vi "Catapult Loop.vi"   [LabVIEW 2015]
uses:
  Robot Global Data.vi
  <vilib>/Rock Robotics/WPI/Solenoid/Deprecated/WPI_SolenoidSetBool.vi
types:
  T1 = typedef "Dashboard Control Data.ctl" = cluster{"Encoder Control":T2, "Steer PID output":cluster{"output high":dbl, "output low":dbl}, " Steer PID gains":cluster{"proportional gain (Kc)":dbl, "integral time (Ti, min)":dbl, "derivative time (Td, min)":dbl}, "Drivetrain Settings":T3, "Vision Packet":T4, "Dashboard Drivetrain Command":T5, "Info/Command Cluster":T7, "Ball Vision Packet":T8, "Intake Presets":T10, "Intake Encoder Control":T12, "Climb Presets":T13, "Goal Output Range":cluster{"output high":dbl, "output low":dbl}, "Enabled Systems":T14, "Auton Presets":T15, "Pressure M":dbl, "Pressure B":dbl, "Vision Timeout":dbl, "Auto-Shift":T16, "Catapult Setpoints":T17}
  T2 = typedef "Encoder Control.ctl" = cluster{"Right Tick Constant":dbl, "Left Tick Constant":dbl, "Reset?":bool, "Y Dist":cluster{"PID gains":cluster{"proportional gain (Kc)":dbl, "integral time (Ti, min)":dbl, "derivative time (Td, min)":dbl}}, "Y Stop Thresh":dbl, "Y Stop Speed":dbl}
  T3 = typedef "Drivetrain Settings.ctl" = cluster{"Gyro Tolerance":dbl, "Throttle Ramp (ms)":dbl, "Kv":dbl, "Ka":dbl, "Feed Forward P":dbl, "Feed Forward D":dbl, "Goal Vision PID gains":cluster{"proportional gain (Kc)":dbl, "integral time (Ti, min)":dbl, "derivative time (Td, min)":dbl}, "Goal Detection Window":dbl, "Creep Rate":dbl, "Vision Throttle Threshold":dbl, "Min Turn Output":dbl, "Left Batter Angle":dbl, "Right Batter Angle":dbl}
  T4 = typedef "Goal Vision Packet.ctl" = cluster{"Distance":dbl, "Center X":dbl, "Center Y":dbl, "Found Target?":bool, "Robot Center":dbl, "Angle":dbl}
  T5 = typedef "Dashboard Drivetrain Command.ctl" = cluster{"Drivetrain Vision":T6}
  T6 = typedef "Drivetrain Vision.ctl" = cluster{"Goal Window":dbl, "Ball Window":dbl}
  T7 = typedef "Ball Tracking Command Cluster.ctl" = cluster{"Distance to Ball":dbl, "Desired Angle":dbl, "Command":enum16{"Turn to Ball", "Turn to Angle", "Get Distance"}, "Pixels from Center":dbl}
  T8 = typedef "Ball Vision Packet.ctl" = cluster{"Ball Detected?":bool, "Distance to Ball":dbl, "Desired Angle":dbl, "Pixels from Center":dbl, "Tracking mode":T9}
  T9 = typedef "Tracking Mode.ctl" = enum16{"Turn to Ball", "Turn to Angle"}
  T10 = typedef "Intake Presets.ctl" = cluster{"Intake Speed":dbl, "Outake Speed":dbl, "Low Height":dbl, "Half Height":dbl, "High Idle Height":dbl, "Angle Speed":dbl, "Angle Tolerance":dbl, "Encoder Scale":dbl, "Load Height":dbl, "Output Range":T11, "Rotation Power Max/Min":dbl, "MaxCurrent":dbl, "Intake Trip Time":dbl, "Idle Height":dbl, "Max Height":dbl, "Reset Encoders?":bool, "PID gains":cluster{"proportional gain (Kc)":dbl, "integral time (Ti, min)":dbl, "derivative time (Td, min)":dbl}, "Intake Stop Delay":u32, "Settle Time":dbl, "Settle Wait Time":dbl, "Pull Up Delay":dbl}
  T11 = typedef "Drivetrain Output Range.ctl" = cluster{"output high":dbl, "output low":dbl}
  T12 = typedef "IntakeEcoderControl.ctl" = cluster{"Arm Tick Constant":dbl, "Reset?":bool, "Y Dist":cluster{"PID gains":cluster{"proportional gain (Kc)":dbl, "integral time (Ti, min)":dbl, "derivative time (Td, min)":dbl}}, "Y Stop Thresh":dbl, "Y Stop Speed":dbl}
  T13 = typedef "Climb Presets.ctl" = cluster{"Pull Power":dbl, "Extend Power":dbl}
  T14 = typedef "Enabled Systems.ctl" = cluster{"Shoot":bool, "Intake":bool, "DT":bool, "Gyro":bool, "100ms":bool, "US":bool}
  T15 = typedef "Autonomous Presets.ctl" = cluster{"Pitch Limit":dbl, "Roll Limit":dbl, "Start Position":dbl, "Cross Position":dbl}
  T16 = typedef "Auto Shift Cluster.ctl" = cluster{"Delay":dbl, "Speed Thresh":dbl, "Upshift Accel":dbl, "Upshift Throttle":dbl, "Upshift Throttle Accel":dbl, "Downshift Throttle":dbl, "Downshift Throttle Accel":dbl, "Pressure Threshold":dbl}
  T17 = typedef "Catapult Presets.ctl" = cluster{"Intake Danger Height":dbl, "Ball Security Delay ":dbl, "High PSI Minimum":dbl, "Shot Finish Delay":dbl, "Low PSI Minimum":dbl, "Idle Ball Security Wait ":dbl}
  T18 = typedef "Catapult Command Cluster.ctl" = cluster{"States":T19, "Mode":T20, "Override IR":bool, "Shoot Mode":T21, "Ball Loaded?":bool, "High Pressure?":bool, "Shoot?":bool, "Flashlight ":bool}
  T19 = typedef "Catapult Auto Commands.ctl" = enum16{"Idle", "Warmup", "Shoot"}
  T20 = typedef "Catapult Modes.ctl" = enum16{"Auto"}
  T21 = typedef "Shoot Mode.ctl" = enum16{"Outer", "Batter"}
  T22 = typedef "WPI_DigitalInputDevRef.ctl" = cluster{"DevStatus":errorcluster, "DIO Channel":T23}
  T23 = typedef "FPGA_DIOChannel.ctl" = enum8{"DIO 0", "DIO 1", "DIO 2", "DIO 3", "DIO 4", "DIO 5", "DIO 6", "DIO 7", "DIO 8", "DIO 9", "DIO MXP 0", "DIO MXP 1", "DIO MXP 2", "DIO MXP 3", "DIO MXP 4", "DIO MXP 5", "DIO MXP 6", "DIO MXP 7", "DIO MXP 8", "DIO MXP 9", "DIO MXP 10", "DIO MXP 11", "DIO MXP 12", "DIO MXP 13", "DIO MXP 14", "DIO MXP 15", "Invalid"}
  T24 = typedef "WPI_RelayDevRef.ctl" = cluster{"DevStatus":errorcluster, "Relay Channel":T25, "Relay Direction":T26}
  T25 = typedef "FPGA_DIORelayChannel.ctl" = enum8{"Relay 0", "Relay 1", "Relay 2", "Relay 3", "Invalid"}
  T26 = typedef "WPI_RelayDirection.ctl" = enum16{"Both directions", "Forward only", "Reverse only"}
  T27 = typedef "Catapult State.ctl" = enum16{"Idle", "Warmup", "Shoot"}
  T28 = typedef "Catapult Status Cluster.ctl" = cluster{"Shoot? ":bool, "Mode":T20, "States":T19, "Shoot Mode":T21, "Override IR ":bool, "Ball Loaded? ":bool, "High Pressure?":bool, "Enough Pressure? ":enum16{"NO ", "Low Pressure", "High Pressure "}, "high 1":bool, "high 2 ":bool, "high 3":bool, "high 4":bool, "Jank Boi":bool, "Ball Security":bool, "Flashlight ":bool}
  T29 = typedef "WPI_SolenoidDevRef.ctl" = cluster{"DevStatus":errorcluster, "Pneumatics Control Module":u8, "Forward Solenoid Channel":T30, "Reverse Solenoid Channel":T30}
  T30 = typedef "WPI_SolenoidChannel.ctl" = enum8{"Solenoid 0", "Solenoid 1", "Solenoid 2", "Solenoid 3", "Solenoid 4", "Solenoid 5", "Solenoid 6", "Solenoid 7", "Invalid"}
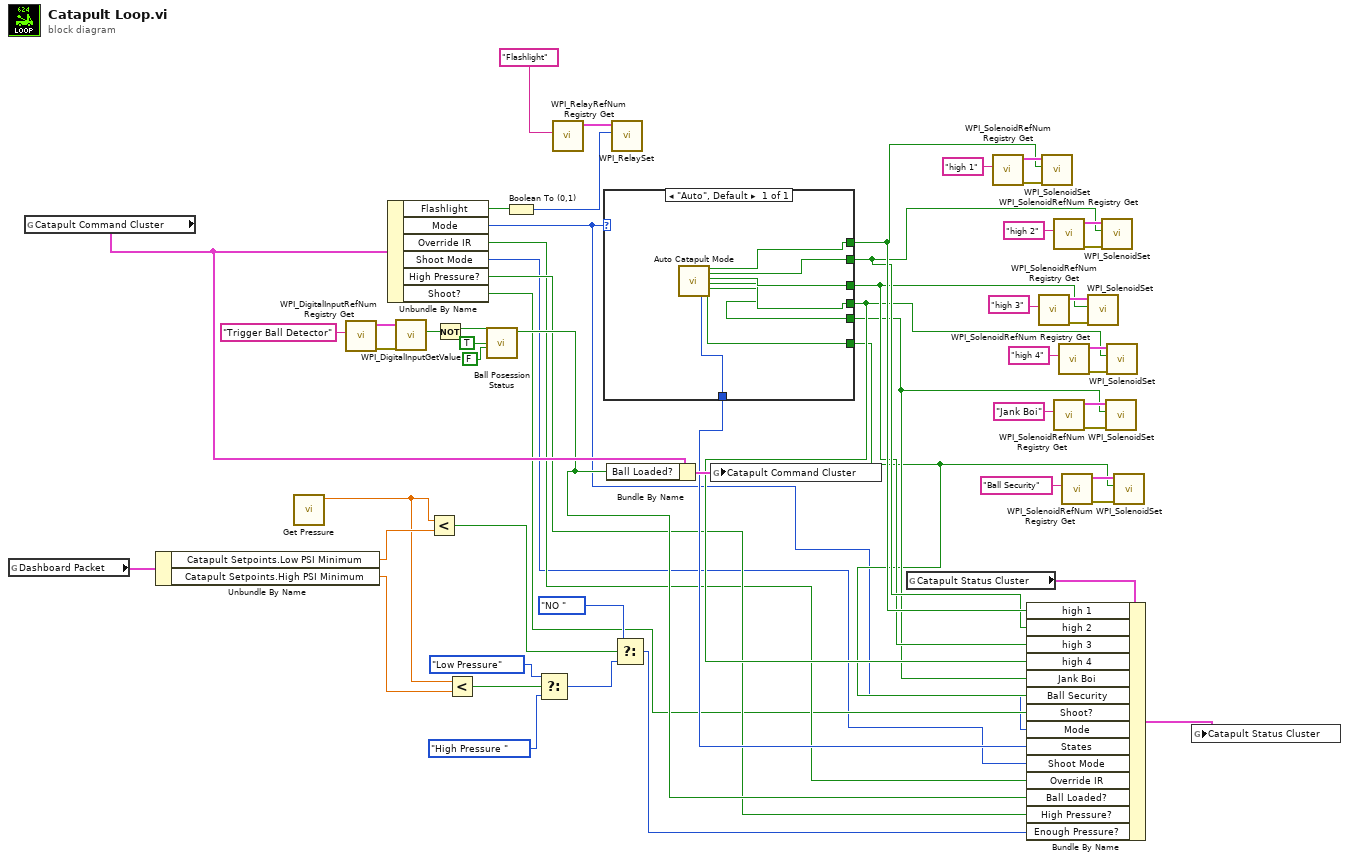
[diagram p0: block diagram]
diagram:
  n1 = global read "Robot Global Data.vi" "Dashboard Packet"() -> (w28:T1)
  n2 = global read "Robot Global Data.vi" "Catapult Command Cluster"() -> (w32:T18)
  n3 = Unbundle By Name(w28) -> ("Catapult Setpoints.Low PSI Minimum"=w27:dbl, "Catapult Setpoints.High PSI Minimum"=w12:dbl)
  n4 = call "Get Pressure.vi"() -> ("Pressure"=w13:dbl)  [unwired: 10 in, 1 out]
  n5 = call <vilib>:"WPI_DigitalInputRefNum Registry Get.vi"("refnum name"="Trigger Ball Detector") -> ("error out"=w44:errorcluster, "DigitalInputDevRef"=w43:T22)  [unwired: 9 in]
  n6 = Unbundle By Name(w32) -> ("Flashlight"=w3:bool, "Mode"=w6:T20, "Override IR"=w8:bool, "Shoot Mode"=w5:T21, "High Pressure?"=w9:bool, "Shoot?"=w7:bool)
  n7 = call <vilib>:"WPI_DigitalInputGetValue.vi"("error in (no error)"=w44, "DigitalInputDevRef"=w43) -> ("Value"=w40:bool)  [unwired: 7 in, 2 out]
  n8 = Less?(x=w13, y=w27) -> (x < y?=w26:bool)
  n9 = Not(x=w40) -> (.not. x?=w39:bool)
  n10 = Less?(x=w13, y=w12) -> (x < y?=w24:bool)
  n11 = call "Ball Posession Status.vi"("Logical Exit?"=FALSE, "Using Sensor?"=TRUE, "Sensor"=w39) -> ("Ball Posessed?"=w10:bool)  [unwired: 8 in]
  n12 = Boolean To (0,1)(Boolean=w3) -> (0, 1=w2:i16)
  n13 = Select(t=enum16{"NO ", "Low Pressure", "High Pressure "}."Low Pressure" ("Enough Pressure?"), s=w24, f=enum16{"NO ", "Low Pressure", "High Pressure "}."High Pressure " ("Enough Pressure?")) -> (s? t:f=w14:enum16{"NO ", "Low Pressure", "High Pressure "})
  n14 = call <vilib>:"WPI_RelayRefNum Registry Get.vi"("refnum name"="Flashlight") -> ("RelayDevRef"=w1:T24)  [unwired: 9 in, 1 out]
  n15 = case shown="\"Auto\", Default" w6 {
    tunnel: [w64] -> w22
    tunnel: [w63] -> w21
    tunnel: [w62] -> w20
    tunnel: [w61] -> w19
    tunnel: [w60] -> w18
    tunnel: [w59] -> w17
    tunnel: [w58] -> w16
    frame "Auto", Default {
      n16 = call "Auto Catapult Mode.vi"() -> ("States"=w58:T27, "high 1"=w64:bool, "high 2"=w63:bool, "high 3"=w62:bool, "high 4"=w61:bool, "Jank Boi"=w60:bool, "Ball Security"=w59:bool)  [unwired: 13 in]
    }
  }
  n17 = Bundle By Name(cluster=w32, "Ball Loaded?"=w10) -> (w31:T18)
  n18 = call <vilib>:"WPI_RelaySet.vi"("RelayValue"=w2, "RelayDevRef"=w1) -> ()  [unwired: 8 in, 2 out]
  n19 = Select(t=enum16{"NO ", "Low Pressure", "High Pressure "}."NO " ("Enough Pressure?"), s=w26, f=w14) -> (s? t:f=w15:enum16{"NO ", "Low Pressure", "High Pressure "})
  n20 = global write "Robot Global Data.vi" "Catapult Command Cluster"(w31) -> ()
  n21 = global read "Robot Global Data.vi" "Catapult Status Cluster"() -> (w29:T28)
  n22 = call <vilib>:"WPI_SolenoidRefNum Registry Get.vi"("refnum name"="high 1") -> ("error out"=w50:errorcluster, "SolenoidDevRef"=w49:T29)  [unwired: 9 in]
  n23 = Bundle By Name(cluster=w29, "high 1"=w22, "high 2"=w21, "high 3"=w20, "high 4"=w19, "Jank Boi"=w18, "Ball Security"=w17, "Shoot?"=w7, "Mode"=w6, "States"=w16, "Shoot Mode"=w5, "Override IR"=w8, "Ball Loaded?"=w10, "High Pressure?"=w9, "Enough Pressure?"=w15) -> (w30:T28)
  n24 = call <vilib>:"WPI_SolenoidRefNum Registry Get.vi"("refnum name"="high 3") -> ("error out"=w34:errorcluster, "SolenoidDevRef"=w33:T29)  [unwired: 9 in]
  n25 = call-poly <vilib>:"WPI_SolenoidSet.vi"("error in (no error)"=w50, "Value"=w22, "SolenoidDevRef"=w49) -> ()  [unwired: 7 in, 2 out]
  n26 = call <vilib>:"WPI_SolenoidRefNum Registry Get.vi"("refnum name"="high 2") -> ("error out"=w52:errorcluster, "SolenoidDevRef"=w51:T29)  [unwired: 9 in]
  n27 = call <vilib>:"WPI_SolenoidRefNum Registry Get.vi"("refnum name"="Jank Boi") -> ("error out"=w54:errorcluster, "SolenoidDevRef"=w53:T29)  [unwired: 9 in]
  n28 = call <vilib>:"WPI_SolenoidRefNum Registry Get.vi"("refnum name"="high 4") -> ("error out"=w36:errorcluster, "SolenoidDevRef"=w35:T29)  [unwired: 9 in]
  n29 = call <vilib>:"WPI_SolenoidRefNum Registry Get.vi"("refnum name"="Ball Security") -> ("error out"=w47:errorcluster, "SolenoidDevRef"=w48:T29)  [unwired: 9 in]
  n30 = call-poly <vilib>:"WPI_SolenoidSet.vi"("error in (no error)"=w34, "Value"=w20, "SolenoidDevRef"=w33) -> ()  [unwired: 7 in, 2 out]
  n31 = call-poly <vilib>:"WPI_SolenoidSet.vi"("error in (no error)"=w52, "Value"=w21, "SolenoidDevRef"=w51) -> ()  [unwired: 7 in, 2 out]
  n32 = call-poly <vilib>:"WPI_SolenoidSet.vi"("error in (no error)"=w54, "Value"=w18, "SolenoidDevRef"=w53) -> ()  [unwired: 7 in, 2 out]
  n33 = call-poly <vilib>:"WPI_SolenoidSet.vi"("error in (no error)"=w36, "Value"=w19, "SolenoidDevRef"=w35) -> ()  [unwired: 7 in, 2 out]
  n34 = call-poly <vilib>:"WPI_SolenoidSet.vi"("error in (no error)"=w47, "Value"=w17, "SolenoidDevRef"=w48) -> ()  [unwired: 7 in, 2 out]
  n35 = global write "Robot Global Data.vi" "Catapult Status Cluster"(w30) -> ()
